vi "Browse OPKG Packages.vi"   [LabVIEW 2020, in "examples.lvlib"]
uses:
  examples.lvlib
  <vilib>/Platform/browser.llb/Open URL in Default Browser (string).vi
  common/common.lvlib
panel:
  # "Run this VI to open the web page you can download .ipk files for this toolkit for."
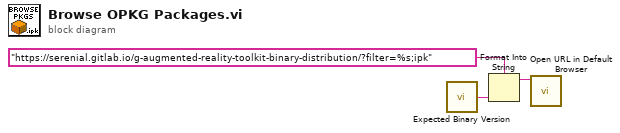
[diagram p0: block diagram]
diagram:
  n1 = call "Expected Binary Version.vi"() -> ("Expected Version"=w2:string)
  n2 = Format Into String(format string="https://serenial.gitlab.io/g-augmented-reality-toolkit-binary-distribution/?filter=%s;ipk", w2) -> (resulting string=w1:string)  [unwired: 2 in, 1 out]
  n3 = call-poly <vilib>:"Open URL in Default Browser.vi"("URL"=w1) -> ()  [unwired: 5 in, 2 out]
